vi "cRIO Module Info.vi"(8 "error in":errorcluster, 10 "Slot (1-N)":u16=1, 11 "Refnum in":refnum<k20>) -> (0 "error out":errorcluster, 2 "cRIO Module Info":T1 {"Product ID" format="%.0x"}, 3 "Refnum out":refnum<k20>)   [LabVIEW 2015, in "RT Management.lvlib" / "Module Detection.lvclass"]
uses:
  Module Detection.lvclass
  Distributed Devices/Controls/DeviceInformation.ctl
  <vilib>/rvi/errors/niLvFpgaAdjustHostInterfaceError.vi
  <vilib>/Utility/error.llb/Error Cluster From Error Code.vi
  <vilib>/rvi/interface/nirviReadWriteControl/nirviReadWriteControl.xnode
  NiFpgaLv.dll
  <vilib>/rvi/interface/Simulation/niFpgaSimulationCallBeginRW.vi
  Distributed Devices/Device.lvclass
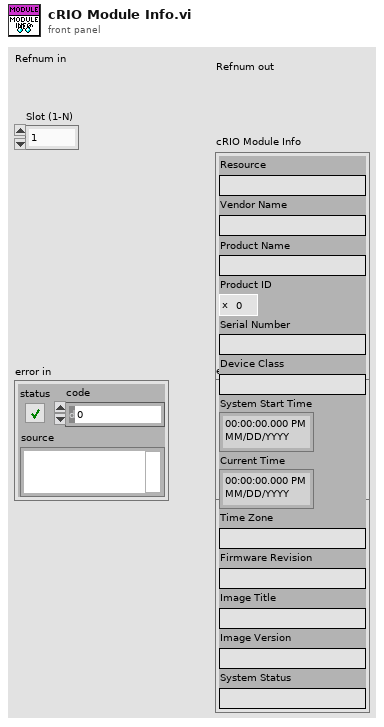
[diagram p1: front panel]
types:
  T1 = typedef "RT Management.lvlib/Device.lvclass/DeviceInformation.ctl" = cluster{"Resource":string, "Vendor Name":string, "Product Name":string, "Product ID":u32, "Serial Number":string, "Device Class":string, "System Start Time":timestamp, "Current Time":timestamp, "Time Zone":string, "Firmware Revision":string, "Image Title":string, "Image Version":string, "System Status":string}
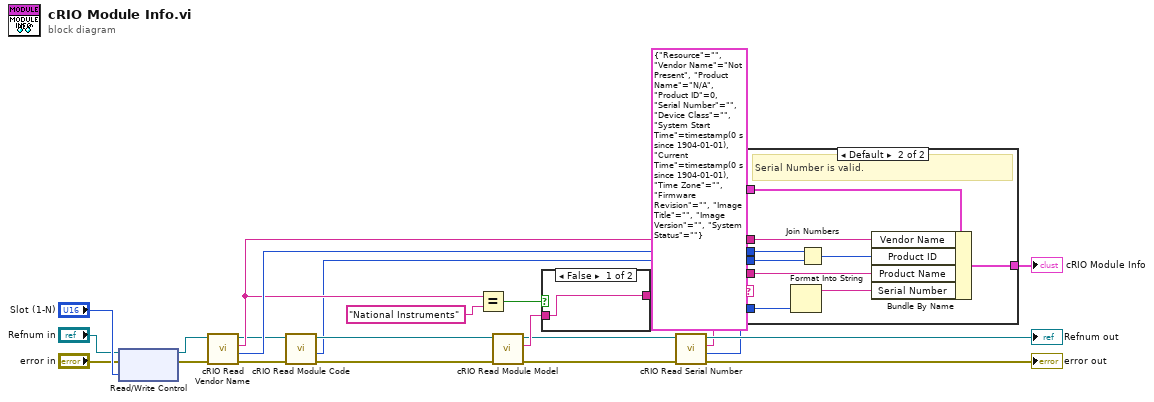
[diagram p0: block diagram]
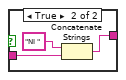
[diagram p2: hidden frame]
diagram:
  n1 = xnode "Read/Write Control"("FPGA VI Reference In"="Refnum in", "error in"="error in", "Module"="Slot (1-N)") -> ("FPGA VI Reference Out"=w22:refnum<k20>, "error out"=w23:errorcluster)
  n2 = call "cRIO Read Vendor Name.vi"("error in"=w23, "Refnum in"=w22) -> ("error out"=w7:errorcluster, "Vendor ID"=w19:u16, "Vendor Name"=w17:string, "Refnum out"=w5:refnum<k20>)  [unwired: 6 in]
  n3 = call "cRIO Read Module Code.vi"("error in"=w7, "Refnum in"=w5) -> ("error out"=w6:errorcluster, "Module ID"=w3:u16, "Refnum out"=w4:refnum<k20>)  [unwired: 6 in, 1 out]
  n4 = Equal?(x=w17, y="National Instruments") -> (x = y?=w15:bool)
  n5 = call "cRIO Read Module Model.vi"("error in"=w6, "Refnum in"=w4) -> ("error out"=w1:errorcluster, "Module Model"=w14:string, "Refnum out"=w2:refnum<k20>)  [unwired: 7 in]
  n6 = case shown="False" w15 {
    tunnel: w14 -> [w25 w27]
    tunnel: [w25 w26] -> w13
    frame False {
    }
    frame True {
      n7 = Concatenate Strings("NI " ("string"), w27) -> (w26:string)
    }
  }
  n8 = call "cRIO Read Serial Number.vi"("error in"=w1, "Refnum in"=w2) -> ("error out"=→"error out":errorcluster, "Serial Number"=w8:u32, "Serial Number String"=w9:string, "Refnum out"=→"Refnum out":refnum<k20>)  [unwired: 6 in]
  n9 = case shown="Default" w9 {
    tunnel: w17 -> [_ w38]
    tunnel: w13 -> [_ w37]
    tunnel: [w29 w36] -> w18
    tunnel: w3 -> [_ w35]
    tunnel: w19 -> [_ w34]
    tunnel: w8 -> [_ w31]
    tunnel: T1 {"Resource"="", "Vendor Name"="Not Present", "Product Name"="N/A", "Product ID"=0, "Serial Number"="", "Device Class"="", "System Start Time"=timestamp(0 s since 1904-01-01), "Current Time"=timestamp(0 s since 1904-01-01), "Time Zone"="", "Firmware Revision"="", "Image Title"="", "Image Version"="", "System Status"=""} ("cRIO Module Info") -> [w29 w32]
    frame "00000000", "FFFFFFFF" {
      # "Empty slot (indicated by invalid Serial Number)."
    }
    frame Default {
      # "Serial Number is valid."
      n10 = Format Into String(w31) -> (resulting string=w30:string)  [unwired: 3 in, 1 out]
      n11 = Join Numbers(hi=w34, lo=w35) -> ((hi.lo)=w33:u32)
      n12 = Bundle By Name(cluster=w32, "Vendor Name"=w38, "Product ID"=w33, "Product Name"=w37, "Serial Number"=w30) -> (w36:T1)
    }
  }
  "cRIO Module Info" <- w18
